vi "network_stream_writer.vi"() -> ()   [LabVIEW 2017]
uses:
  Utility Sub VIs/diode_charts.ctl
  <vilib>/dex/Stream Element Allocation Mode.ctl
  Input Channel Lists/pg_control_physical_channels.ctl
  Input Channel Lists/valve_physical_channels.ctl
  Input Channel Lists/window_heater_physical_channels.ctl
panel:
  in  "data in":string
  in  "notification 2":T1
  in  "notification":T1
  in  "Output":T5={"Pulse Generator Control Physical Channels"={"1000W 1"="Output/port0/line1", "1000W 2"="Output/port0/line2", "1000W 3"="Output/port0/line3", "500W 1"="Output/port0/line4", "250W 1"="Output/port0/line5", "150W 1"="Output/port0/line6", "Counter Line"="cDAQ1Mod1/ctr0", "Direction Line"="cDAQ1Mod1/port0/line1", "USB \nController"=""}, "Proportional Valve Physical Channels"={"Vapor Valve"="cDAQ1Mod3/ao1", "Liquid Valve"="cDAQ1Mod3/ao2", "PG Valve"="cDAQ1Mod3/ao0"}, "Window Heaters Physical Channels"={"On/Off"="cDAQ1Mod4/ao0"}, "Diode Communication"={"URL"="", "Serial"=""}}
  in  "Stop":bool
  # "NI-9401 Counter & DIO (pin) Chart"
  # "Default Pins used by Counter:\n     SRC: P-Gen Counter Timebase, A-input  \n     GATE: P-Gen Trigger, Z-input\n     AUX: B-input \n     OUT: P_Gen Output\nMore info:  Programs»National Instruments»NI-DAQ»NI-DAQmx Key Concepts»Counters"
  # "0"
  # "1"
  # "2"
  # "3"
  # "7 (25)"
  # "6 (23)"
  # "4 (20)"
  # "5 (22)"
  # "3 (19)"
  # "2 (17)"
  # "0 (14)"
  # "1 (16)"
  # "4 (20)"
  # "5 (22)"
  # "6 (23)"
  # "7 (25)"
  # "0 (14)"
  # "1 (16)"
  # "2 (17)"
  # "3 (19)"
  # "COUNTER"
  # "SRC"
  # "GATE"
  # "AUX"
  # "OUT"
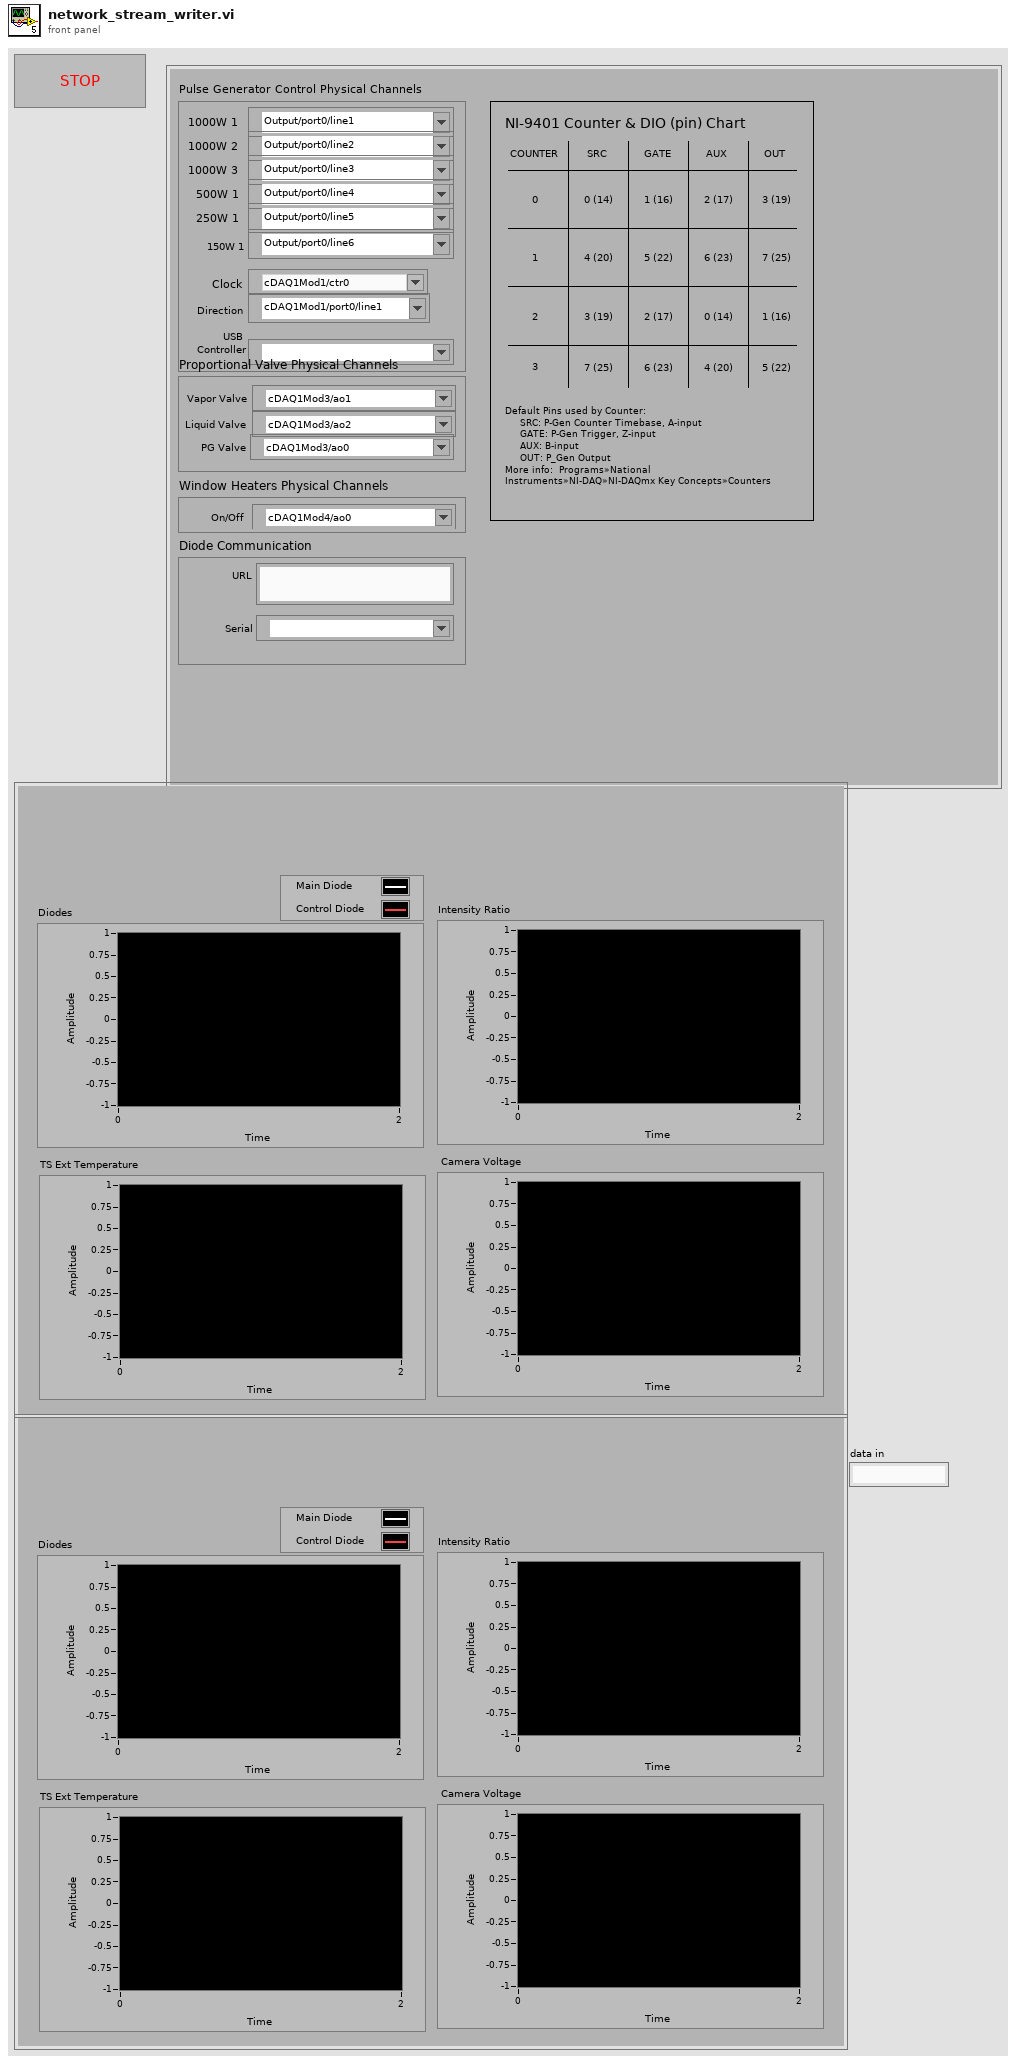
[diagram p1: front panel]
types:
  T1 = cluster{"Diodes":cluster{dbl, dbl}[], "Intensity Ratio":dbl[], "TS Ext Temperature":dbl[], " Camera Voltage":dbl[]}
  T2 = typedef "pg_control_physical_channels.ctl" = cluster{"1000W 1":tag, "1000W 2":tag, "1000W 3":tag, "500W 1":tag, "250W 1":tag, "150W 1":tag, "Counter Line":tag, "Direction Line":tag, "USB \nController":refnum<visa-resource-name>}
  T3 = typedef "valve_physical_channels.ctl" = cluster{"Vapor Valve":tag, "Liquid Valve":tag, "PG Valve":tag}
  T4 = typedef "window_heater_physical_channels.ctl" = cluster{"On/Off":tag}
  T5 = cluster{"Pulse Generator Control Physical Channels":T2, "Proportional Valve Physical Channels":T3, "Window Heaters Physical Channels":T4, "Diode Communication":cluster{"URL":string, "Serial":refnum<visa-resource-name>}}
  T6 = typedef "Stream Element Allocation Mode.ctl" = u32
  T7 = typedef "diode_charts.ctl" = cluster{"Liquid Diodes":cluster{dbl, dbl}, "Liquid Intensity Ratio":dbl, "Vapor Diode":cluster{dbl, dbl}, "Vapor Intensity Ratio":dbl, "TS Window 1 Temperatures":cluster{"Average":dbl, "T Sat [C]":dbl}}
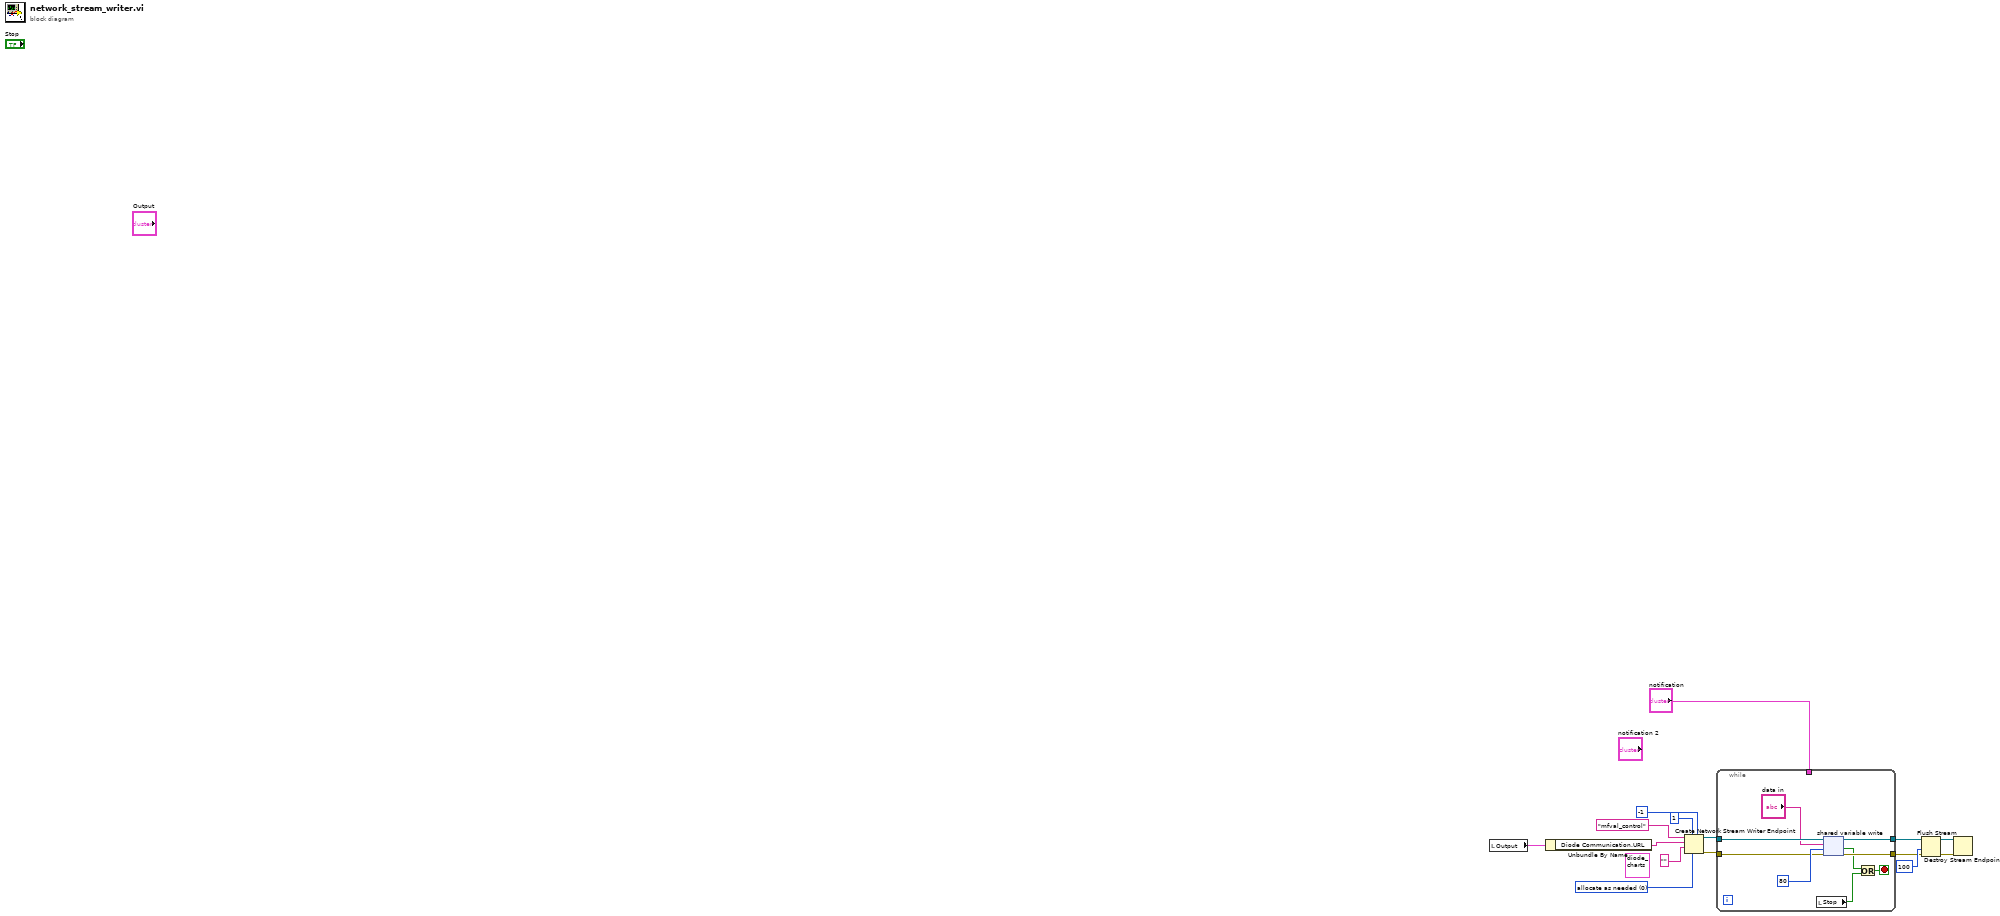
[diagram p0: block diagram]
diagram:
  w12 = T6 0 items=["allocate as needed", "pre-allocate"] ("element allocation mode")
  (unwired) T7 {"Liquid Diodes"={0.0, 0.0}, "Liquid Intensity Ratio"=0.0, "Vapor Diode"={0.0, 0.0}, "Vapor Intensity Ratio"=0.0, "TS Window 1 Temperatures"={"Average"=0.0, "T Sat [C]"=0.0}} ("Diode Charts")
  n1 = local read "Output"() -> (w14:T5)
  n2 = Unbundle By Name(w14) -> ("Diode Communication.URL"=w2:string)
  n3 = Create Network Stream Writer Endpoint(5:-1 ("timeout in ms (-1)"), 6:w12, 7:1 ("writer buffer size"), 9:"", 10:w2, 11:"mfval_control" ("writer name")) -> (0:w4:errorcluster, 3:w5:refnum<k21>)  [unwired: 1 in]
  n4 = while {
    tunnel: w5 -> [w21]
    tunnel: [w23] -> w7
    tunnel: w4 -> [w17]
    tunnel: [w22] -> w6
    tunnel: "notification" -> [_]
    stop <- w20 stop-if-true
    n5 = local read "Stop"() -> (w18:bool)
    n6 = shared-variable-write(w21, w17, "data in", 80 ("timeout ms (-1)")) -> (w23:refnum<k21>, w22:errorcluster, w19:bool)
    n7 = Or(x=w19, y=w18) -> (x .or. y?=w20:bool)
  }
  n8 = Flush Stream(8:w6, 9:100 ("timeout in ms (-1)"), 11:w7) -> (0:w9:errorcluster, 3:w8:refnum<k21>)  [unwired: 1 in, 1 out]
  n9 = Destroy Stream Endpoint(8:w9, 11:w8) -> ()  [unwired: 1 out]
